vi "AnalyzeCornerPosition (SubVI).vi"(4 "Center-only search?":bool, 7 "Placement tolerance [um]":dbl=10.0, 8 "error in (no error)":errorcluster, 9 "Fiducial Template":T2, 10 "Calibration [um/pix]":dbl=0.25, 11 "Refnum in":T2) -> (0 "error out":errorcluster, 1 "Y offset [um]":sgl, 2 "X offset [um]":sgl, 3 "Refnum out":T2, 5 "Offset interpreter":T3)   [LabVIEW 2016]
uses:
  <vilib>/vision/Image Controls.llb/IMAQ Image.ctl
  <vilib>/vision/NI_Vision_Development_Module.lvlib
panel:
  in  "Search Rect":T1={"Left"=0, "Top"=0, "Right"=2147483647, "Bottom"=2147483647, "Rotation"=0.0} {"Rotation" format="%.2f"; "Left" scale=0.0..1024.0; "Right" scale=0.0..1024.0}
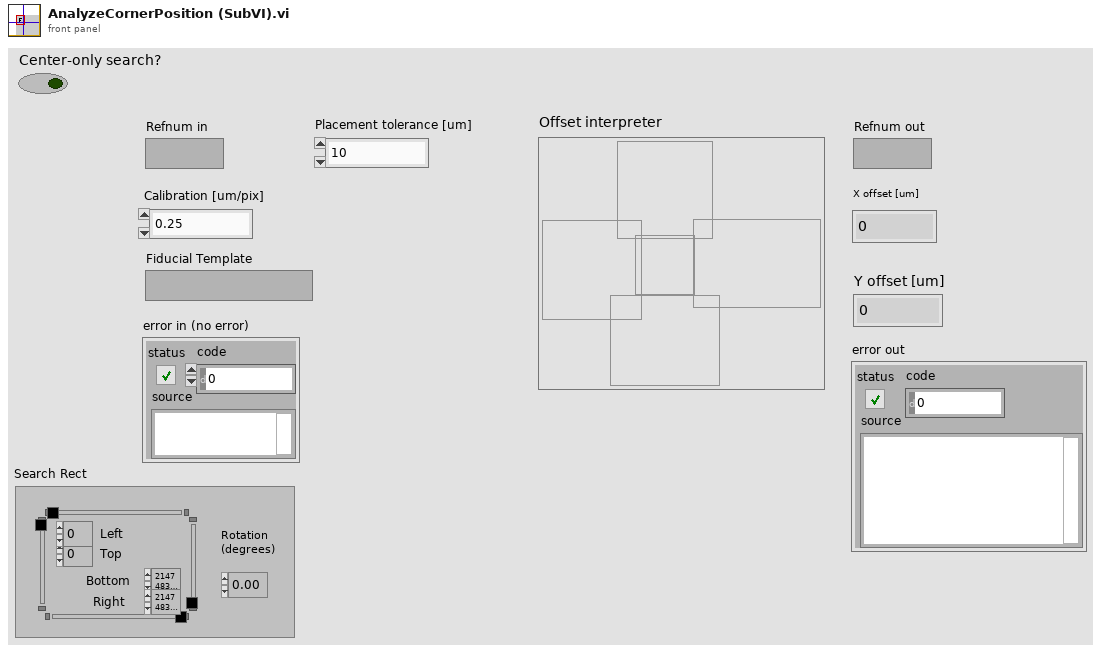
[diagram p1: front panel]
types:
  T1 = typedef "IMAQ Rectangle" = cluster{"Left":i32, "Top":i32, "Right":i32, "Bottom":i32, "Rotation":dbl}
  T2 = typedef "IMAQ Image.ctl" = refnum<image>
  T3 = cluster{"Offset Interpreter - Right":bool, "Offset Interpreter - forward":bool, "Offset Interpreter - backward":bool, "Offset Interpreter - Left":bool, "Placement Confirmation":bool}
  T4 = cluster{"Algorithm":i32, "Number of Matches Requested":i32, "Minimum Match Score":sgl, "SubPixel Accuracy":bool, "Rotation Angle Ranges":cluster{"Start":sgl, "End":sgl}[], "Show Search Area":bool, "Show Result":bool}
  T5 = cluster{"Position":cluster{"x":sgl, "y":sgl}, "Angle":sgl, "Scale":sgl, "Score":sgl, "Bounding Box":cluster{"x":sgl, "y":sgl}[]}[]
  T6 = cluster{"Position":cluster{"x":sgl, "y":sgl}, "Angle":sgl, "Scale":sgl, "Score":sgl, "Bounding Box":cluster{"x":sgl, "y":sgl}[]}
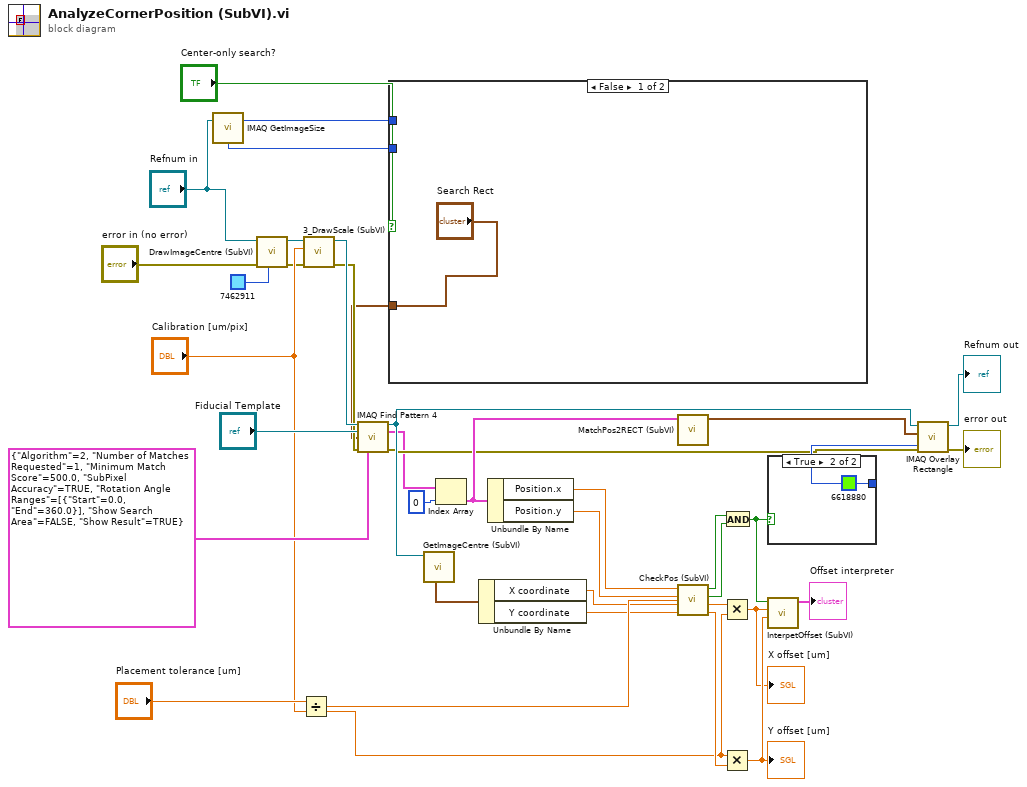
[diagram p0: block diagram]
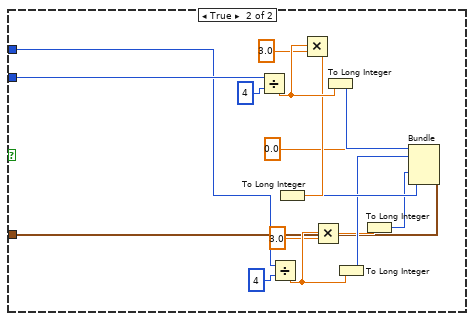
[diagram p2: hidden frame]
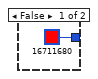
[diagram p3: hidden frame]
diagram:
  n1 = call "IMAQ GetImageSize"("Image"="Refnum in") -> ("Y Resolution"=w1:i32, "X Resolution"=w2:i32)  [unwired: 3 in, 1 out]
  n2 = call "DrawImageCentre (SubVI).vi"("Axis colour"=u32 7462911, "error in (no error)"="error in (no error)", "Refnum in"="Refnum in") -> ("error out"=w6:errorcluster, "Refnum out"=w36:T2)  [unwired: 7 in]
  n3 = Divide(x="Placement tolerance [um]", y="Calibration [um/pix]") -> (x/y=w29:dbl)
  n4 = call "3_DrawScale (SubVI).vi"("um/pix"="Calibration [um/pix]", "Refnum in"=w36) -> ("Refnum out"=w37:T2)  [unwired: 9 in]
  n5 = case shown="False" "Center-only search?" {
    tunnel: ["Search Rect" w42] -> w5
    tunnel: w2 -> [_ w41]
    tunnel: w1 -> [_ w40]
    frame False {
    }
    frame True {
      n6 = Divide(x=w41, y=4) -> (x/y=w52:dbl)
      n7 = Divide(x=w40, y=4) -> (x/y=w47:dbl)
      n8 = Multiply(x=w52, y=3.0) -> (x*y=w50:dbl)
      n9 = To Long Integer(number=w50) -> (32bit integer=w49:i32)
      n10 = Multiply(x=w47, y=3.0) -> (x*y=w44:dbl)
      n11 = To Long Integer(number=w52) -> (32bit integer=w53:i32)
      n12 = To Long Integer(number=w47) -> (32bit integer=w45:i32)
      n13 = To Long Integer(number=w44) -> (32bit integer=w43:i32)
      n14 = Bundle(w53, w45, w49, w43, "y"=0.0) -> (w42:cluster{i32, i32, i32, i32, "y":dbl})  [unwired: 1 in]
    }
  }
  n15 = call "IMAQ Find Pattern 4"("Image"=w37, "Template"="Fiducial Template", "Search Rect"=w5, "error in"=w6, "Settings"=T4 {"Algorithm"=2, "Number of Matches Requested"=1, "Minimum Match Score"=500.0, "SubPixel Accuracy"=TRUE, "Rotation Angle Ranges"=[{"Start"=0.0, "End"=360.0}], "Show Search Area"=FALSE, "Show Result"=TRUE}) -> ("Image Out"=w20:T2, "Matches (pixel)"=w15:T5, "error out"=w17:errorcluster)  [unwired: 4 in, 4 out]
  n16 = call "GetImageCentre (SubVI).vi"("Image in \n(refnum)"=w20) -> ("Centre Point"=w21:cluster{"X coordinate":dbl, "Y coordinate":dbl})  [unwired: 4 in, 4 out]
  n17 = Index Array(array=w15, index=0) -> (element=w25:T6)
  n18 = Unbundle By Name(w21) -> ("X coordinate"=w22:dbl, "Y coordinate"=w23:dbl)
  n19 = Unbundle By Name(w25) -> ("Position.x"=w9:sgl, "Position.y"=w8:sgl)
  n20 = call "MatchPos2RECT (SubVI).vi"("Match element"=w25) -> ("Rectangle"=w14:cluster{"x":sgl, "y":sgl, dbl, dbl})  [unwired: 10 in]
  n21 = call "CheckPos (SubVI).vi"("x"=w9, "y"=w8, "true x"=w22, "true y"=w23, "variation tolerance"=w29) -> ("pass x coordinate"=w18:bool, "pass y coordinate"=w19:bool, "delta X"=w26:sgl, "delta Y"=w27:sgl)  [unwired: 2 in]
  n22 = Multiply(x=w26, y="Calibration [um/pix]") -> (x*y=w33:dbl)
  "X offset [um]" <- w33
  n23 = Multiply(x="Calibration [um/pix]", y=w27) -> (x*y=w34:dbl)
  "Y offset [um]" <- w34
  n24 = And(x=w18, y=w19) -> (x .and. y?=w32:bool)
  n25 = case shown="True" w32 {
    tunnel: [u32 16711680 ("Color") u32 6618880 ("Color")] -> w24
    frame False {
    }
    frame True {
    }
  }
  n26 = call "InterpetOffset (SubVI).vi"("Y offset"=w34, "X offset"=w33, "Good position"=w32) -> ("Offset interpreter"=→"Offset interpreter":T3)  [unwired: 8 in]
  n27 = call "IMAQ Overlay Rectangle"("Color"=w24, "error in (no error)"=w17, "Rectangle"=w14, "Image"=w20) -> ("error out"=→"error out":errorcluster, "Image Out"=→"Refnum out":T2)  [unwired: 6 in]
